vi "Create ErrorHandler.vi"(8 "error in (no error)":errorcluster, 11 "IWampMessage":refnum<class "IWampMessage.lvclass">) -> (0 "error out":errorcluster, 3 "IErrorHandler out":refnum<class "IErrorHandler.lvclass">)   [LabVIEW 2020, in "wamplv.lvlib"]
uses:
  wamplv.lvlib
  SerialisedMessages/IWampMessage/IWampMessage.lvclass
  SerialisedMessages/JSONMessage/WampMessage JSON.lvclass
  SerialisedMessages/MsgPackMessage/WampMessage MsgPack.lvclass
  ErrorHandler JSON/ErrorHandler JSON.lvclass
  ErrorHandler MsgPack/ErrorHandler MsgPack.lvclass
  C:/local/wamplv/Private/Requests/MessageReceivedHandlers/Error/IAbortOrErroHandler/IAbortOrErrorHandler.lvclass
  C:/local/wamplv/Private/Requests/IInternalMessage/IInternalMessage.lvclass
  C:/local/wamplv/Private/Requests/MessageReceivedHandlers/IErrorHandler/IErrorHandler.lvclass
  C:/local/wamplv/Private/Requests/MessageReceivedHandlers/Error/ErrorHandler JSON/ErrorHandler JSON.lvclass
  C:/local/wamplv/Private/Requests/MessageReceivedHandlers/IJsonMessageHandler/IJsonMessageHandler.lvclass
  C:/local/wamplv/Private/Requests/MessageReceivedHandlers/Error/ErrorHandler MsgPack/ErrorHandler MsgPack.lvclass
  C:/local/wamplv/Private/Requests/MessageReceivedHandlers/IMsgPackMessageHandler/IMsgPackMessageHandler.lvclass
  IErrorHandler/IErrorHandler.lvclass
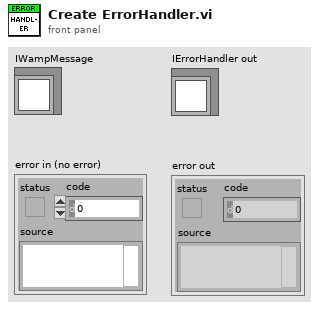
[diagram p1: front panel]
types:
  T1 = typedef "wamplv.lvlib/WAMP Client.lvclass/Serialisation.ctl" = enum16{"JSON", "MessagePack"}
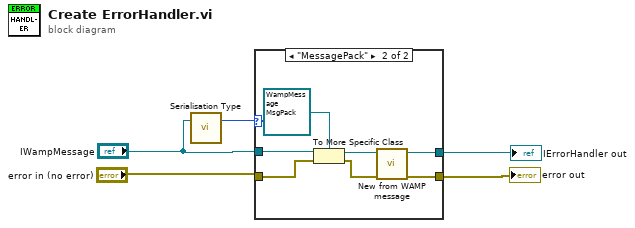
[diagram p0: block diagram]
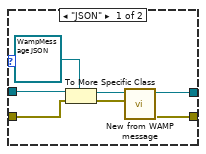
[diagram p2: hidden frame]
diagram:
  n1 = call-dynamic "Serialisation Type.vi"("IWampMessage in"="IWampMessage") -> ("Serialisation Type"=w5:T1)  [unwired: 2 in]
  n2 = case shown="\"MessagePack\"" w5 {
    tunnel: "IWampMessage" -> [w12 w19]
    tunnel: "error in (no error)" -> [w10 w18]
    tunnel: [w6 w13] -> w1
    tunnel: [w7 w14] -> w2
    frame "JSON" {
      n3 = To More Specific Class(target class=refnum<class "WampMessage JSON.lvclass"> refnum ("wamplv.lvlib:JSONMessage.lvclass"), reference=w12, error in=w10) -> (specific class reference=w9:refnum<class "WampMessage JSON.lvclass">, error out=w8:errorcluster)
      n4 = call "New from WAMP message.vi"("error in (no error)"=w8, "wamplv.lvlib:JSONMessage.lvclass"=w9) -> ("error out"=w6:errorcluster, "ErrorHandler JSON out"=w7:refnum<class "ErrorHandler JSON.lvclass">)  [unwired: 7 in, 1 out]
    }
    frame "MessagePack" {
      n5 = To More Specific Class(target class=refnum<class "WampMessage MsgPack.lvclass"> refnum ("wamplv.lvlib:MsgPackMessage.lvclass"), reference=w19, error in=w18) -> (specific class reference=w16:refnum<class "WampMessage MsgPack.lvclass">, error out=w15:errorcluster)
      n6 = call "New from WAMP message.vi"("error in (no error)"=w15, "WampMessage MsgPack"=w16) -> ("error out"=w13:errorcluster, "ErrorHandler MsgPack out"=w14:refnum<class "ErrorHandler MsgPack.lvclass">)  [unwired: 7 in, 1 out]
    }
  }
  "error out" <- w1
  "IErrorHandler out" <- w2
